vi "Add.vi"(1 "B":dbl, 2 "A":dbl) -> (0 "A+B":dbl)   [LabVIEW 2018]
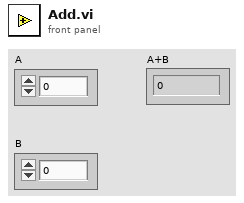
[diagram p1: front panel]
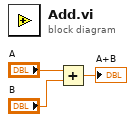
[diagram p0: block diagram]
diagram:
  n1 = Add(x="A", y="B") -> (x+y=→"A+B":dbl)
